vi "Read Laser State.vi"(8 "error in (no error)":errorcluster, 11 "Laser Ethernet Cabinet in":refnum<class "Laser Ethernet Cabinet.lvclass">) -> (0 "error out":errorcluster, 2 "Laser State":T1, 3 "Laser Ethernet Cabinet out":refnum<class "Laser Ethernet Cabinet.lvclass">)   [LabVIEW 2023, in "Laser Ethernet Cabinet.lvclass"]
uses:
  Laser Ethernet Cabinet.lvclass
  Laser Ethernet Cabinet.lvclass/Laser Ethernet Cabinet.ctl
  log_status.ctl
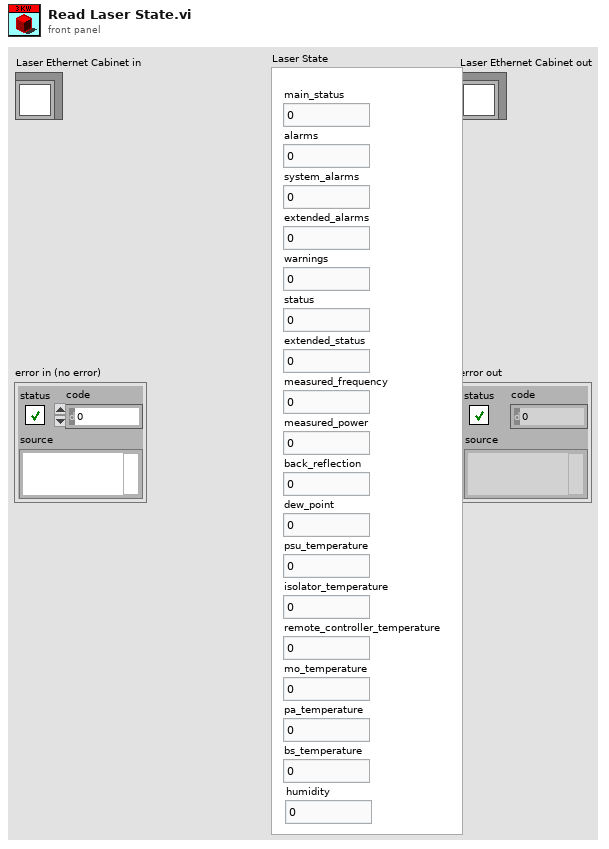
[diagram p1: front panel]
types:
  T1 = typedef "Laser Ethernet Cabinet.lvclass/log_status.ctl" = cluster{"main_status":u32, "alarms":u32, "system_alarms":u32, "extended_alarms":u32, "warnings":u32, "status":u32, "extended_status":u32, "measured_frequency":sgl, "measured_power":sgl, "back_reflection":sgl, "dew_point":sgl, "psu_temperature":sgl, "isolator_temperature":sgl, "remote_controller_temperature":sgl, "mo_temperature":sgl, "pa_temperature":sgl, "bs_temperature":sgl, "humidity":sgl}
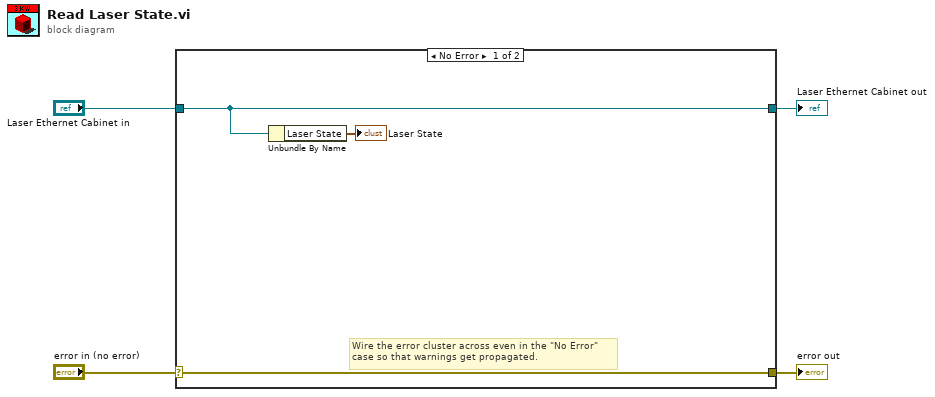
[diagram p0: block diagram]
diagram:
  n1 = case shown="No Error" "error in (no error)" {
    selector: "error in (no error)" -> [w7 w9]
    tunnel: [w7 w9] -> w3
    tunnel: [w6 w8] -> w1
    tunnel: "Laser Ethernet Cabinet in" -> [w6 w8]
    frame No Error {
      # "Wire the error cluster across even in the \"No Error\"\ncase so that warnings get propagated."
      n2 = Unbundle By Name(w6) -> ("Laser State"=→"Laser State":T1)
    }
    frame Error {
    }
  }
  "error out" <- w3
  "Laser Ethernet Cabinet out" <- w1
